vi "HEWH Agilent Create Channel Array.vi"(8 "Error In":errorcluster, 9 "Agilent Raw Cluster Array":T1, 10 "Agilent Calibrated Cluster Array":T1, 11 "Channel Array In":string[](array[string])) -> (0 "Error Out":errorcluster, 1 "Agilent Raw Cluster Array Out":T1, 2 "Agilent Calibrated Cluster Array Out":T1, 3 "Channel Array Out":string[](array[string]))   [LabVIEW 2019]
uses:
  Type Definitions/HEWH Agilent Cluster.ctl
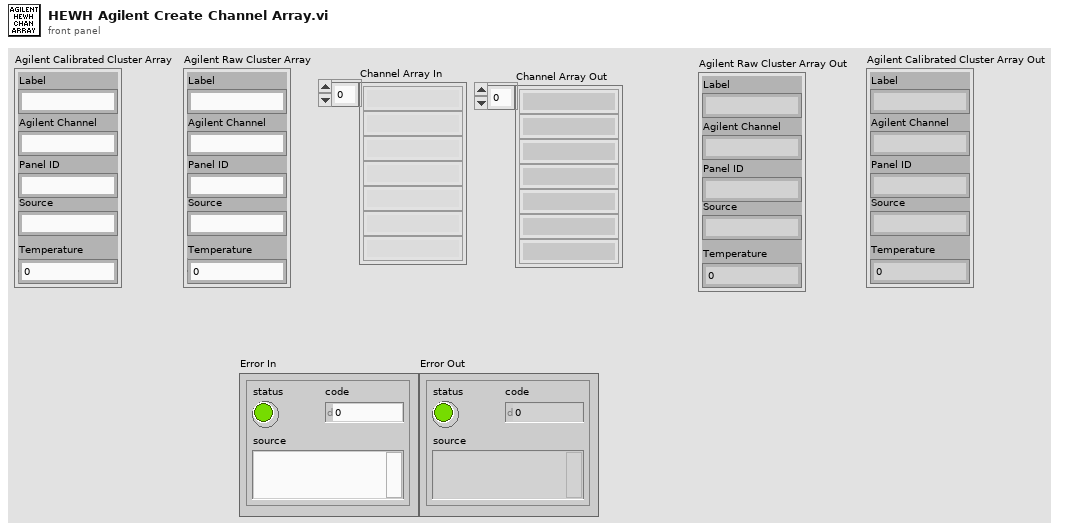
[diagram p1: front panel]
types:
  T1 = typedef "HEWH Agilent Cluster.ctl" = cluster{"Label":string, "Agilent Channel":string, "Panel ID":string, "Source":string, "Temperature":dbl}
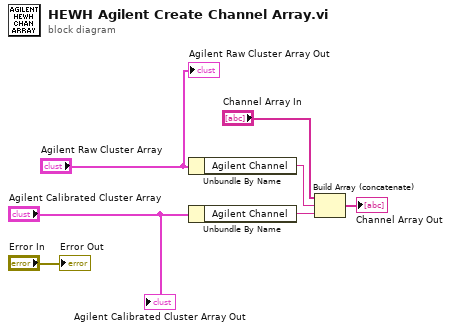
[diagram p0: block diagram]
diagram:
  n1 = Unbundle By Name("Agilent Raw Cluster Array") -> ("Agilent Channel"=w3:string)
  n2 = Unbundle By Name("Agilent Calibrated Cluster Array") -> ("Agilent Channel"=w1:string)
  n3 = Build Array (concatenate)("Channel Array In", w3, w1) -> (→"Channel Array Out":string[])
  "Agilent Raw Cluster Array Out" <- "Agilent Raw Cluster Array"
  "Error Out" <- "Error In"
  "Agilent Calibrated Cluster Array Out" <- "Agilent Calibrated Cluster Array"
